vi "Parse Hierarchy Table Row.vi"(8 "Error in":errorcluster caption="Error in (no error)", 11 "Rows Array JSON":string) -> (0 "Error out":errorcluster, 3 "data":T1)   [LabVIEW 2018]
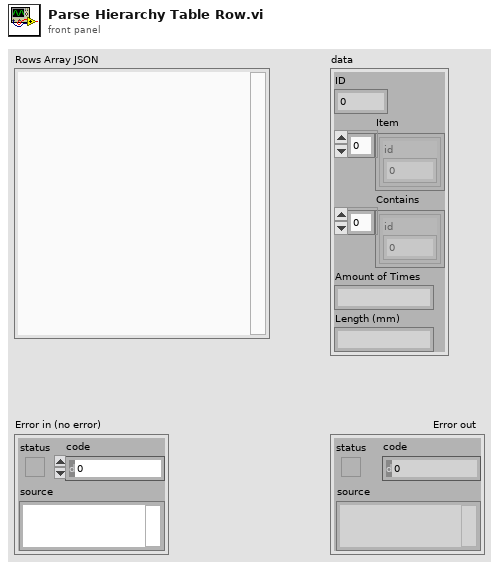
[diagram p1: front panel]
types:
  T1 = cluster{"ID":i32, "Item":cluster{"id":i32}[], "Contains":cluster{"id":i32}[], "Amount of Times":string, "Length (mm)":string}
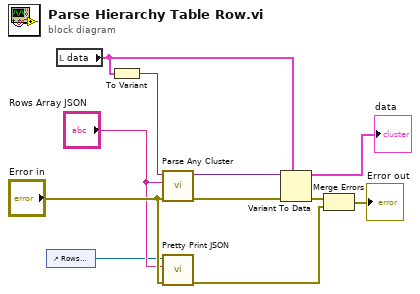
[diagram p0: block diagram]
diagram:
  n1 = control-ref of="Rows Array JSON"() -> (w1:refnum<vi>)
  n2 = local read "data"() -> (w9:T1)
  n3 = To Variant(anything=w9) -> (Variant=w6:variant)
  n4 = call "Parse Any Cluster.vi"("error in (no error)"="Error in", "JSON In"="Rows Array JSON", "Cluster in"=w6) -> ("error out"=w8:errorcluster, "Cluster out"=w11:variant)  [unwired: 7 in]
  n5 = call "Pretty Print JSON.vi"("error in (no error)"="Error in", "JSON in"="Rows Array JSON", "String in"=w1) -> ("error out"=w5:errorcluster)  [unwired: 8 in]
  n6 = Variant To Data(error in=w8, type=w9, Variant=w11) -> (data=→"data":T1, error out=w7:errorcluster)
  n7 = Merge Errors(w7, w5) -> (→"Error out":errorcluster)
